vi "Read Waveforms Subset from Buffer.vi"(0 "Waveforms (N Ch)":refnum<class "Waveforms (N Ch).lvclass">, 7 "timestamp":timestamp format="%<%H:%M:%S%6u\n%x>T", 9 "block length":i32, 11 "error in (no error)":errorcluster) -> (3 "subset status":T1(ring), 4 "Waveforms (N Ch)":refnum<class "Waveforms (N Ch).lvclass">, 6 "waveforms subset":waveform(dbl)[](array[waveform]), 8 "actual timestamp":timestamp format="%<%H:%M:%S%6u\n%x>T", 10 "actual length":i32, 14 "end of buffer":bool, 15 "error out":errorcluster)   [LabVIEW 2017, in "Waveforms (N Ch).lvclass"]
doc: "Use this VI to access the waveform data from the Waveforms (N Ch) object. This VI also returns the timestamp of the waveform data as well as the number of samples. This VI returns empty data until all requested data is available."
uses:
  <vilib>/addons/_NISVFA/_Shared subVIs/Data Objects/Waveforms (DBL)/Waveforms (N Ch).lvclass
  C:/Program Files (x86)/National Instruments/LabVIEW 2017/vi.lib/addons/_NISVFA/_Shared subVIs/Data Objects/Data/Data.lvclass
  <vilib>/addons/_NISVFA/_Shared subVIs/Data Objects/Data/Data.lvclass/Data.ctl
  <vilib>/addons/_NISVFA/_Shared subVIs/Data Objects/Waveforms (DBL)/Waveforms (N Ch).lvclass/Waveforms (N Ch).ctl
  <vilib>/addons/_NISVFA/_Shared subVIs/Common/svc_Copy Waveform Subset (Index).vi
  <vilib>/addons/_NISVFA/_Shared subVIs/Common/sv_Get NI Property Name String.vi
  <vilib>/addons/_NISVFA/_Shared subVIs/Common/svc_Copy Array Subset (Index).vi
  <vilib>/addons/_NISVFA/_Shared subVIs/Common/svc_Coerce Index and Length.vi
  <vilib>/addons/_NISVFA/_Shared subVIs/Common/svc_Conditional Merge Error.vi
  <vilib>/addons/_NISVFA/_Shared subVIs/Data Objects/Data/Data.lvclass
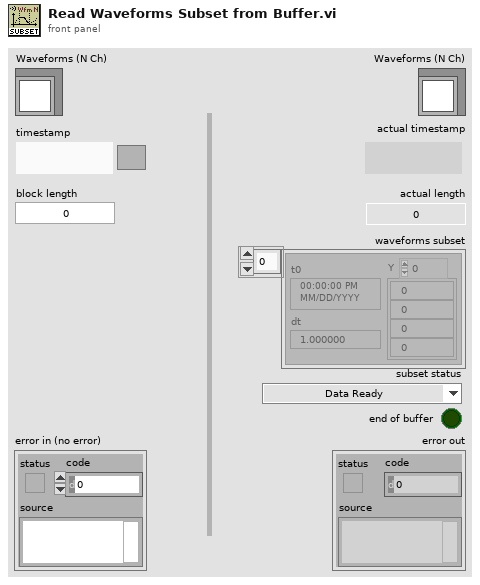
[diagram p1: front panel]
types:
  T1 = enum16{"Data Ready", "First Sample Not Yet Available", "Last Sample Not Yet Available", "Data No Longer Available"}
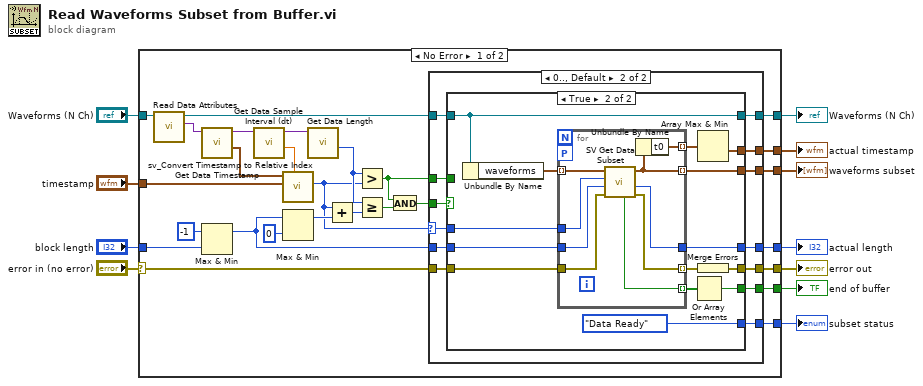
[diagram p0: block diagram]
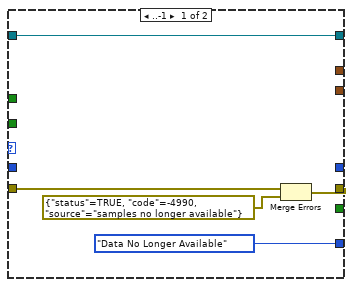
[diagram p2: hidden frame]
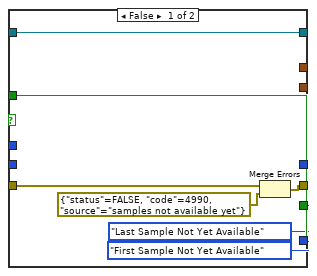
[diagram p3: hidden frame]
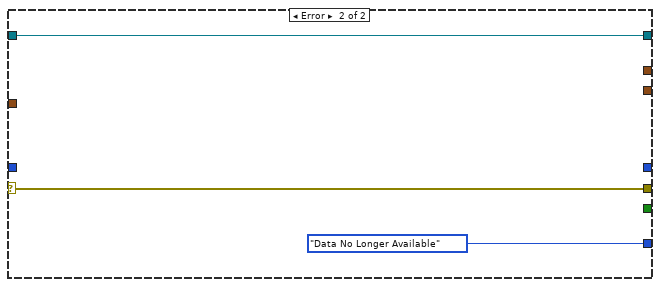
[diagram p4: hidden frame]
diagram:
  n1 = case shown="No Error" "error in (no error)" {
    selector: "error in (no error)" -> [w37 w90]
    tunnel: [w30 w90] -> w5
    tunnel: [w13 w91] -> w9
    tunnel: "Waveforms (N Ch)" -> [w38 w91]
    tunnel: "timestamp" -> [w31 _]
    tunnel: [w29 _] -> w7
    tunnel: "block length" -> [w25 _]
    tunnel: [w36 _] -> w4
    tunnel: [w28 _] -> w3
    tunnel: [w27 T1."Data No Longer Available"] -> w2
    tunnel: [w24 _] -> w1
    frame No Error {
      n2 = call <vilib>:"Read Data Attributes.vi"("Data in"=w38) -> ("data attributes"=w35:variant, "Data out"=w14:refnum<class "Waveforms (N Ch).lvclass">)  [unwired: 8 in, 1 out]
      n3 = call <vilib>:"Get Data Timestamp.vi"("variant in"=w35) -> ("timestamp"=w32:timestamp, "variant out"=w34:variant)  [unwired: 9 in]
      n4 = Max & Min(x=-1 ("y"), y=w25) -> (max(x,y)=w18:i32)  [unwired: 1 out]
      n5 = call <vilib>:"Get Data Sample Interval (dt).vi"("variant in"=w34) -> ("dt [s]"=w33:dbl, "variant out"=w23:variant)  [unwired: 9 in]
      n6 = call <vilib>:"sv_Convert Timestamp to Relative Index.vi"("waveform dt"=w33, "timestamp"=w31, "waveform timestamp"=w32) -> ("Y index"=w12:i32)  [unwired: 8 in]
      n7 = Max & Min(x=w18, y=0 ("x")) -> (max(x,y)=w20:i32)  [unwired: 1 out]
      n8 = call <vilib>:"Get Data Length.vi"("variant in"=w23) -> ("number of samples"=w15:i32)  [unwired: 9 in, 1 out]
      n9 = Add(x=w12, y=w20) -> (x+y=w21:i32)
      n10 = Greater?(x=w15, y=w12) -> (0:w16:bool)
      n11 = Greater Or Equal?(x=w15, y=w21) -> (x >= y?=w22:bool)
      n12 = And(x=w16, y=w22) -> (x .and. y?=w17:bool)
      n13 = case shown="0.., Default" w12 {
        selector: w12 -> [_ w48]
        tunnel: w37 -> [w41 w56]
        tunnel: [_ w55] -> w36
        tunnel: [w40 w54] -> w30
        tunnel: [_ w53] -> w29
        tunnel: [_ w52] -> w28
        tunnel: [T1."Data No Longer Available" ("subset status") w51] -> w27
        tunnel: w18 -> [_ w50]
        tunnel: [_ w49] -> w24
        tunnel: w17 -> [_ w46]
        tunnel: w16 -> [_ w47]
        tunnel: w14 -> [w39 w45]
        tunnel: [w39 w44] -> w13
        frame ..-1 {
          n14 = Merge Errors(w41, errorcluster {"status"=TRUE, "code"=-4990, "source"="samples no longer available"} ("error in (no error)")) -> (w40:errorcluster)
        }
        frame 0.., Default {
          n15 = case shown="True" w46 {
            tunnel: w56 -> [w61 w79]
            tunnel: [_ w77] -> w55
            tunnel: [w60 w76] -> w54
            tunnel: [_ w67] -> w53
            tunnel: [_ w75] -> w52
            tunnel: [w59 T1."Data Ready" ("subset status")] -> w51
            tunnel: w50 -> [_ w74]
            tunnel: [TRUE ("end of buffer") w73] -> w49
            tunnel: w48 -> [_ w70]
            tunnel: w47 -> [w63 _]
            tunnel: w45 -> [w58 w66]
            tunnel: [w58 w66] -> w44
            frame False {
              n16 = Merge Errors(w61, errorcluster {"status"=FALSE, "code"=4990, "source"="samples not available yet"} ("error in (no error)")) -> (w60:errorcluster)
              n17 = Select(t=T1."Last Sample Not Yet Available" ("subset status"), s=w63, f=T1."First Sample Not Yet Available" ("subset status")) -> (s? t:f=w59:T1)
            }
            frame True {
              n18 = Unbundle By Name(w66) -> ("waveforms"=w68:waveform(dbl)[])
              n19 = for {
                tunnel: w74 -> [w88]
                tunnel: w79 -> [w87]
                tunnel: [w86] -> w72 mode=indexing
                tunnel: [w85] -> w78 mode=indexing
                workers-P: _ -> [_]
                tunnel: [w84] -> w75
                tunnel: w70 -> [w83]
                tunnel: [w82] -> w71 mode=indexing
                tunnel: [w81] -> w67 mode=indexing
                tunnel: w68 -> [w80] mode=indexing
                n20 = call-poly <vilib>:"SV Get Data Subset.vi"("error in (no error)"=w87, "length (-1 = all)"=w88, "start index (0)"=w83, "waveform in"=w80) -> ("error out"=w86:errorcluster, "actual length"=w84:i32, "waveform subset"=w81:waveform(dbl), "end reached"=w82:bool)  [unwired: 3 in, 1 out]
                n21 = Unbundle By Name(w81) -> ("t0"=w85:timestamp)
              }
              n22 = Or Array Elements(Boolean array=w71) -> (logical OR=w73:bool)
              n23 = Array Max & Min(array=w78) -> (min value=w77:timestamp)  [unwired: 3 out]
              n24 = Merge Errors(w72) -> (w76:errorcluster)
            }
          }
        }
      }
    }
    frame Error {
    }
  }
  "error out" <- w5
  "Waveforms (N Ch)" <- w9
  "waveforms subset" <- w7
  "end of buffer" <- w1
  "actual timestamp" <- w4
  "actual length" <- w3
  "subset status" <- w2
